vi "Settings_Vindow.vi"(11 "Data":T2={"Core"={"Current VI Reference"=refnum, "Close Panel on Exit?"=FALSE, "Start Timestmap"="", "Status His"="", "Active"=FALSE, "Exit"=FALSE, "Assignment structure"=""}, "Sample ID"="", "Cam"={"Cam"="", "Connected"=FALSE, "Sim Image"=FALSE, "Save pictures"=FALSE}, "UR"={"PC_IP"="", "Remote port"=0, "UR_IP"="", "connection ID"=refnum, "Connected"=FALSE, "Sim UR signal"=FALSE, "UR Ready"=FALSE, "Ready fail"=0.0}, "Sample data"={"Insects taken from current picture"=0, "Number of insects in pick-up area"=0, "Object data"={"Object CoM X"=0.0, "Object CoM Y"=0.0, "Corrected Object orientation"=0.0, "Object length"=0.0, "Z, Height"=0.0}, "Raw Particle Measurements"=[], "Insect-data-array"=[], "Sorted Particle Measurements"=[], "Insects to pick this round"=0, "Picking array"=[], "Pixels Measurements"=[], "Tool1 to pick"=0}, "Images"={"Image"=refnum, "Image Timestamp"="", "Boarder Image"=refnum, "Vision A. Image"=refnum}, "Reshake"=0, "Settings"={"Number to try and pick"=0, "Last few"=0, "Z_Zero"=0.0, "Tool switch size"=0.0, "X-Zero"=0.0, "Y-Zero"=0.0, "Small or XL"=0.0, "Tool1-Height"=12.0, "Tool2-Height"=12.0, "Ignore small"=12.0, "Time to Whait"=25.0}, "Assignment"={"Executing Assignment"="", "Task"="", "Tool"="", "Specimen to pick"=0, "GO"=FALSE}, "Return reason"=""} {"Sample data"."Object data"."Z, Height" format="%#_13g"}) -> (2 "OK":bool, 3 "output cluster":T2={"Core"={"Current VI Reference"=refnum, "Close Panel on Exit?"=FALSE, "Start Timestmap"="", "Status His"="", "Active"=FALSE, "Exit"=FALSE, "Assignment structure"=""}, "Sample ID"="", "Cam"={"Cam"="", "Connected"=FALSE, "Sim Image"=FALSE, "Save pictures"=FALSE}, "UR"={"PC_IP"="192.168.0.15", "Remote port"=30002, "UR_IP"="192.168.0.10", "connection ID"=refnum, "Connected"=FALSE, "Sim UR signal"=FALSE, "UR Ready"=FALSE, "Ready fail"=0.0}, "Sample data"={"Insects taken from current picture"=0, "Number of insects in pick-up area"=0, "Object data"={"Object CoM X"=0.0, "Object CoM Y"=0.0, "Corrected Object orientation"=0.0, "Object length"=0.0, "Z, Height"=0.0}, "Raw Particle Measurements"=[], "Insect-data-array"=[], "Sorted Particle Measurements"=[], "Insects to pick this round"=0, "Picking array"=[], "Pixels Measurements"=[], "Tool1 to pick"=0}, "Images"={"Image"=refnum, "Image Timestamp"="", "Boarder Image"=refnum, "Vision A. Image"=refnum}, "Reshake"=0, "Settings"={"Number to try and pick"=8, "Last few"=4, "Z_Zero"=0.1, "Tool switch size"=2.0, "X-Zero"=-35.0, "Y-Zero"=406.0, "Small or XL"=12.0, "Tool1-Height"=12.0, "Tool2-Height"=12.0, "Ignore small"=12.0, "Time to Whait"=25.0}, "Assignment"={"Executing Assignment"="", "Task"="", "Tool"="", "Specimen to pick"=0, "GO"=FALSE}, "Return reason"=""} {"Sample data"."Object data"."Z, Height" format="%#_13g"})   [LabVIEW 2024]
uses:
  SRS/controls/IHS_JKI.ctl
  <vilib>/userDefined/High Color/IMAQdx.ctl
  <vilib>/vision/Image Controls.llb/IMAQ Image.ctl
panel:
  in  "Inputs":T1={"Last few"=0, "Try to pick"=8, "Y-offset"=0.0, "X-offset"=0.0, "Z_height"=0.0, "Small or XL"=12.0, "Tool switch size"=2.0, "UR_IP"="192.168.0.10", "Remote port"=30002, "PC_IP"="192.168.0.15", "Tool1-Height"=0.1, "Tool2-Height"=0.0, "Ignore small"=12.0, "Time to whait"=25.0}
  in  "Cancel Button":bool
  in  "OK Button":bool
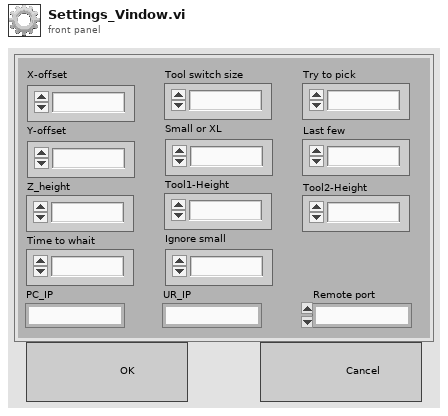
[diagram p1: front panel]
types:
  T1 = cluster{"Last few":i32, "Try to pick":i32, "Y-offset":dbl, "X-offset":dbl, "Z_height":dbl, "Small or XL":dbl, "Tool switch size":dbl, "UR_IP":string, "Remote port":u16, "PC_IP":string, "Tool1-Height":dbl, "Tool2-Height":dbl, "Ignore small":dbl, "Time to whait":dbl}
  T2 = typedef "IHS_JKI.ctl" = cluster{"Core":cluster{"Current VI Reference":refnum<vi>, "Close Panel on Exit?":bool, "Start Timestmap":string, "Status His":string, "Active":bool, "Exit":bool, "Assignment structure":string}, "Sample ID":string, "Cam":cluster{"Cam":T3, "Connected":bool, "Sim Image":bool, "Save pictures":bool}, "UR":cluster{"PC_IP":string, "Remote port":u16, "UR_IP":string, "connection ID":refnum<k5>, "Connected":bool, "Sim UR signal":bool, "UR Ready":bool, "Ready fail":dbl}, "Sample data":cluster{"Insects taken from current picture":i32, "Number of insects in pick-up area":i32, "Object data":cluster{"Object CoM X":dbl, "Object CoM Y":dbl, "Corrected Object orientation":dbl, "Object length":dbl, "Z, Height":dbl}, "Raw Particle Measurements":dbl[][], "Insect-data-array":string[][], "Sorted Particle Measurements":dbl[][], "Insects to pick this round":i32, "Picking array":dbl[][], "Pixels Measurements":dbl[][], "Tool1 to pick":i32}, "Images":cluster{"Image":T4, "Image Timestamp":string, "Boarder Image":T4, "Vision A. Image":T4}, "Reshake":i32, "Settings":cluster{"Number to try and pick":i32, "Last few":i32, "Z_Zero":dbl, "Tool switch size":dbl, "X-Zero":dbl, "Y-Zero":dbl, "Small or XL":dbl, "Tool1-Height":dbl, "Tool2-Height":dbl, "Ignore small":dbl, "Time to Whait":dbl}, "Assignment":cluster{"Executing Assignment":string, "Task":string, "Tool":string, "Specimen to pick":i32, "GO":bool}, "Return reason":string}
  T3 = typedef "IMAQdx.ctl" = refnum<k21>
  T4 = typedef "IMAQ Image.ctl" = refnum<image>
  T5 = cluster{"Number to try and pick":i32, "Last few":i32, "Z_Zero":dbl, "Tool switch size":dbl, "X-Zero":dbl, "Y-Zero":dbl, "Small or XL":dbl, "Tool1-Height":dbl, "Tool2-Height":dbl, "Ignore small":dbl, "Time to Whait":dbl}
  T6 = cluster{"PC_IP":string, "Remote port":u16, "UR_IP":string, "connection ID":refnum<k5>, "Connected":bool, "Sim UR signal":bool, "UR Ready":bool, "Ready fail":dbl}
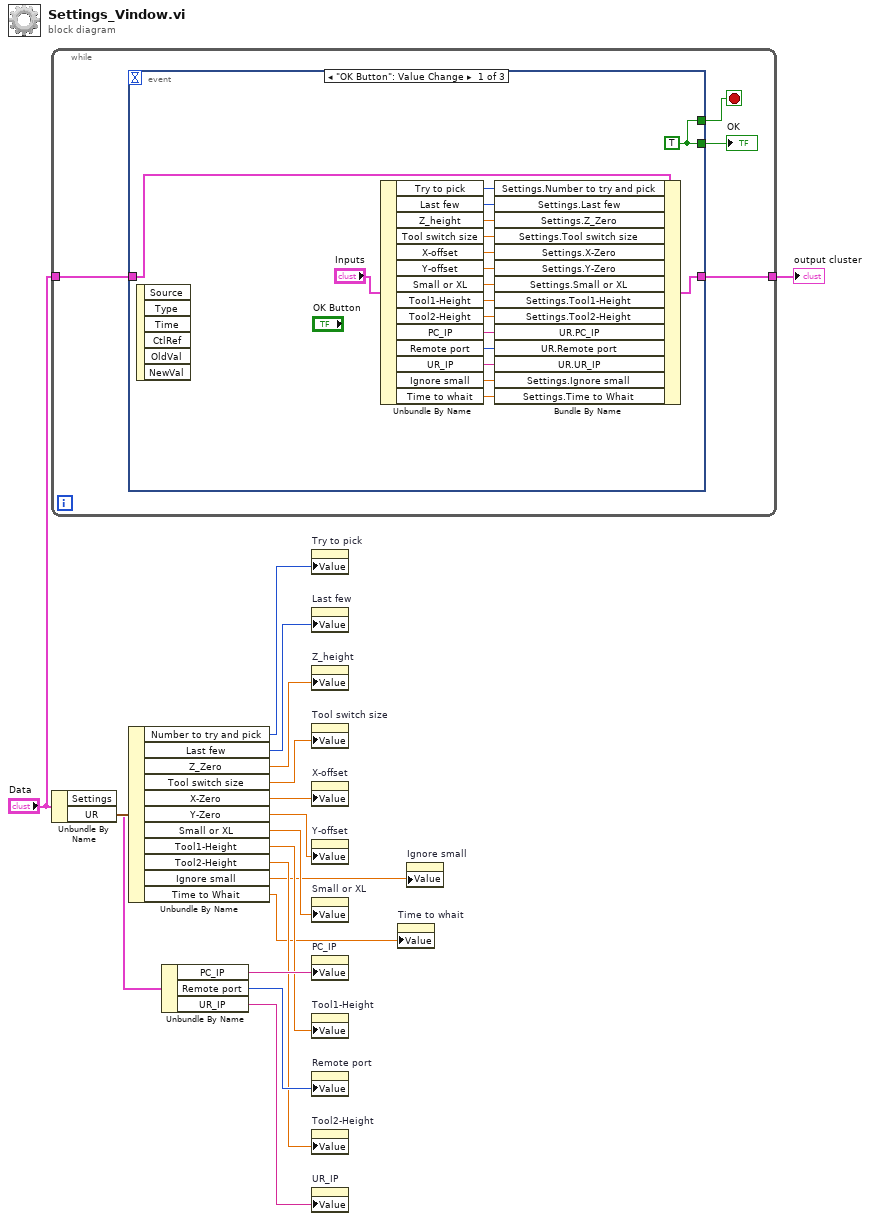
[diagram p0: block diagram]
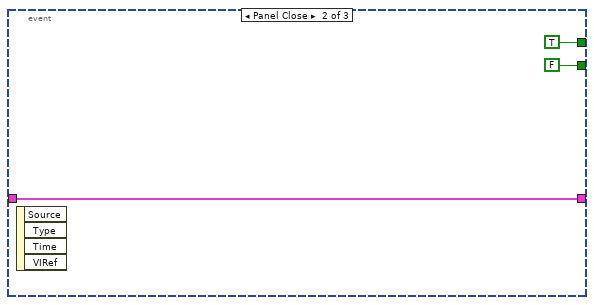
[diagram p2: hidden frame]
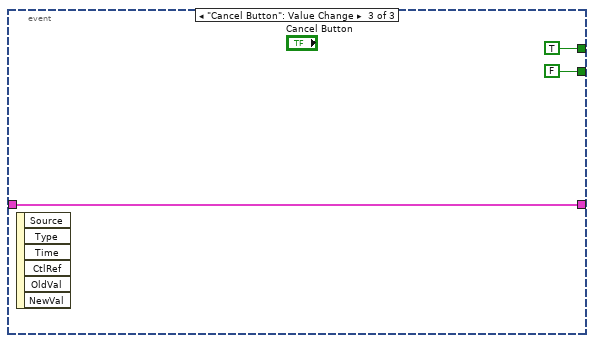
[diagram p3: hidden frame]
diagram:
  n1 = while {
    tunnel: "Data" -> [w19]
    tunnel: [w20] -> w15
    stop <- w21 stop-if-true
    n2 = event shown="[0] \"OK Button\": Value Change" {
      selector: _ -> [_ _ _]
      dyn-events: _ -> [_ _ _]
      timeout: _ -> [_ _ _]
      tunnel: [w40 FALSE FALSE] -> w22
      tunnel: [w40 TRUE TRUE] -> w21
      tunnel: [w27 w41 w44] -> w20
      tunnel: w19 -> [w39 w41 w44]
      event "OK Button": Value Change {
        w40 = TRUE
        n3 = event-data() -> ()  [unwired: 1 in, 6 out]
        n4 = Unbundle By Name("Inputs") -> ("Try to pick"=w37:i32, "Last few"=w36:i32, "Z_height"=w35:dbl, "Tool switch size"=w34:dbl, "X-offset"=w33:dbl, "Y-offset"=w32:dbl, "Small or XL"=w31:dbl, "Tool1-Height"=w30:dbl, "Tool2-Height"=w25:dbl, "PC_IP"=w26:string, "Remote port"=w29:u16, "UR_IP"=w28:string, "Ignore small"=w24:dbl, "Time to whait"=w23:dbl)
        n5 = Bundle By Name(cluster=w39, "Settings.Number to try and pick"=w37, "Settings.Last few"=w36, "Settings.Z_Zero"=w35, "Settings.Tool switch size"=w34, "Settings.X-Zero"=w33, "Settings.Y-Zero"=w32, "Settings.Small or XL"=w31, "Settings.Tool1-Height"=w30, "Settings.Tool2-Height"=w25, "UR.PC_IP"=w26, "UR.Remote port"=w29, "UR.UR_IP"=w28, "Settings.Ignore small"=w24, "Settings.Time to Whait"=w23) -> (w27:T2)
      }
      event Panel Close {
        n6 = event-data() -> ()  [unwired: 1 in, 4 out]
      }
      event "Cancel Button": Value Change {
        n7 = event-data() -> ()  [unwired: 1 in, 6 out]
      }
    }
    "OK" <- w22
  }
  "output cluster" <- w15
  n8 = Unbundle By Name("Data") -> ("Settings"=w17:T5, "UR"=w16:T6)
  n9 = Unbundle By Name(w17) -> ("Number to try and pick"=w9:i32, "Last few"=w8:i32, "Z_Zero"=w12:dbl, "Tool switch size"=w11:dbl, "X-Zero"=w14:dbl, "Y-Zero"=w13:dbl, "Small or XL"=w10:dbl, "Tool1-Height"=w4:dbl, "Tool2-Height"=w3:dbl, "Ignore small"=w2:dbl, "Time to Whait"=w1:dbl)
  n10 = Unbundle By Name(w16) -> ("PC_IP"=w5:string, "Remote port"=w7:u16, "UR_IP"=w6:string)
  n11 = property on="Try to pick" class="DigNum (strict)"("Value"=w9) -> ()  [unwired: 2 in, 2 out]
  n12 = property on="Last few" class="DigNum (strict)"("Value"=w8) -> ()  [unwired: 2 in, 2 out]
  n13 = property on="Z_height" class="DigNum (strict)"("Value"=w12) -> ()  [unwired: 2 in, 2 out]
  n14 = property on="Tool switch size" class="DigNum (strict)"("Value"=w11) -> ()  [unwired: 2 in, 2 out]
  n15 = property on="X-offset" class="DigNum (strict)"("Value"=w14) -> ()  [unwired: 2 in, 2 out]
  n16 = property on="Y-offset" class="DigNum (strict)"("Value"=w13) -> ()  [unwired: 2 in, 2 out]
  n17 = property on="Small or XL" class="DigNum (strict)"("Value"=w10) -> ()  [unwired: 2 in, 2 out]
  n18 = property on="PC_IP" class="Str"("Value"=w5) -> ()  [unwired: 2 in, 2 out]
  n19 = property on="Tool1-Height" class="DigNum (strict)"("Value"=w4) -> ()  [unwired: 2 in, 2 out]
  n20 = property on="Remote port" class="DigNum (strict)"("Value"=w7) -> ()  [unwired: 2 in, 2 out]
  n21 = property on="Tool2-Height" class="DigNum (strict)"("Value"=w3) -> ()  [unwired: 2 in, 2 out]
  n22 = property on="UR_IP" class="Str"("Value"=w6) -> ()  [unwired: 2 in, 2 out]
  n23 = property on="Time to whait" class="DigNum (strict)"("Value"=w1) -> ()  [unwired: 2 in, 2 out]
  n24 = property on="Ignore small" class="DigNum (strict)"("Value"=w2) -> ()  [unwired: 2 in, 2 out]
